vi "FPGA_RAPS.vi"(8 "error in":errorcluster) -> (0 "error out":errorcluster)   [LabVIEW 2010]
uses:
  fpgaVIsAndControls/DDS_board_init_cluster.ctl
  common_typedefs/channels_cluster.ctl
  fpgaVIsAndControls/FPGA_parameters_cluster.ctl
  common_typedefs/gate_parameters_cluster.ctl
  fpgaVIsAndControls/derived_values.ctl
  fpgaVIsAndControls/scan_point_cluster.ctl
  fpgaVIsAndControls/DDS_board_values_cluster.ctl
  fpgaVIsAndControls/synthesizer_point_cluster.ctl
  <vilib>/Platform/TimedLoop/XDataNode/XDataNode.xnode
  <vilib>/Platform/TimedLoop/XDataNode/timing_clust.ctl
  <vilib>/Platform/TimedLoop/XDataNode/nitl_modes.ctl
  <vilib>/Platform/TimedLoop/XDataNode/wakeup.ctl
  <vilib>/eio/EIONode/EIONode.xnode
  <vilib>/rvi/eio/nirviEIOImplementation/nirviEIOImplementation.xnode
  <vilib>/rvi/eio/common/nirviEmuClasses.ctl
  <vilib>/rvi/eio/nirviErrorMerge/nirviErrorMerge.xnode
  <vilib>/rvi/DataTransferAndStorage/Container/XNode/niFpgaContainer.xnode
  <vilib>/rvi/DataTransferAndStorage/Container/Common/niFpgaContainerMethod.ctl
  <vilib>/rvi/DataTransferAndStorage/Container/Common/niFpgaTransferTypeControl.ctl
  <vilib>/rvi/eio/common/nirviEmuTemplateMethod_noerrors.vi
  <vilib>/rvi/eio/common/nirviEmuTemplateMethod_errors.vi
  <vilib>/rvi/interface/RandomDataEmulation/nirviRandomDataFPGAFIFO.vi
  <vilib>/rvi/interface/RandomDataEmulation/niFpgaRandomDataHandleErrors.vi
  <vilib>/rvi/FIFO/Fifo_Resource/nirvififoEmulationSetSize.vi
  <vilib>/rvi/DataTransferAndStorage/Container/Common/niFpgaContainerGetUniqueNameForEmu.vi
  <vilib>/Platform/TimedLoop/XDataNode/XDNodeRunTimeDep.lvlib
panel:
  in  "shall acquisition start clocks?":bool
  in  "run clock 3":bool
  in  "run clock 2":bool
  in  "run clock 1":bool
  out "current memory pointer":i32
  in  "current raps point":T1
  out "current write address":u32
  in  "button:storePoint":bool
  out "current synthesizer point":T2
  out "current frequency point":T3
  out "current raps point":T1
  in  "point package size":u8=1
  out "derived values":T4={"AOD half bandwidth_x"=17500000.0, "AOD half bandwidth_y"=17500000.0, "x-point bandwidth"=10.0, "y-point bandwidth"=10.0} {"y-point bandwidth" format="%.28g"; "x-point bandwidth" format="%.28g"; "AOD half bandwidth_y" format="%.14g"; "AOD half bandwidth_x" format="%.14g"}
  out "next pixel?":bool
  in  "integration delay (iterations)":u32
  in  "integration delay (pixels)":u32
  in  "first pixel black?":bool
  in  "gate 1":T5
  in  "gate 2":T5
  in  "gate 3":T5
  out "clock 2 state":bool
  out "clock 1 state":bool
  out "clock 3 state":bool
  out "acquiring?":bool
  in  "in triggered mode?":bool
  in  "stop at FIFO overflow?":bool
  in  "converter box version":i16=1 min=1 max=2
  out "reset out":bool
  in  "ra trajectory pixels\n(data/pixels transfered)":u32=65535
  in  "amp comp":bool
  in  "inverse?":T6(ring)
  in  "OSK select":bool=TRUE
  in  "FPGA parameters":T7={"AOD Bandwidth_x (Hz)"=34000000.0, "AOD Bandwidth_y (Hz)"=34000000.0, "sin Phi"=0.0, "cos Phi"=1.0, "Bandwidth for LUTs (256pts)"=0.9999999999854481, "AOD_Amplitude in"=3400, "AOD center frequ. (Hz)_x"=94000000.0, "AOD center frequ. (Hz)_y"=94000000.0, "x offset (Hz)"=0.0, "y offset (Hz)"=0.0} {"AOD center frequ. (Hz)_y" format="%.14g"; "AOD center frequ. (Hz)_x" format="%.14g"; "cos Phi" format="%.35g"; "sin Phi" format="%.35g"}
  out "integrated pixel values":T8
  in  "maximum bit depth":i8=16
  in  "pixel iterations":u32=40
  in  "equilibration iterations":u32=200
  out "data read":T8
  in  "channel offsets":T8
  in  "number of pixels":i64=-1
  out "FIFO_DMA0 full?":bool
  out "current pixel no.":i64
  in  "acquire?":bool caption="Acquire?"
  in  "Stop complete VI":bool caption="Stop"
  in  "reset in":bool caption="Reset"
  in  "DDS board initialization parameters":T9={"Bypass PLL"=FALSE, "PLL Range"=TRUE, "Update Clock"=FALSE, "Triangle "=FALSE, "SDO Active"=FALSE, "LSB First"=FALSE, "OSK Int"=FALSE, "Output Shaped Keying Enable"=TRUE, "Bypass Sinc"=FALSE, "Digital Part"=TRUE, "OutPut DAC"=TRUE, "Control DAC"=TRUE, "Comparator"=FALSE, "Modus"=0, "Multiplier Value"=15} {"Modus" scale=0.0..4.0}
  # "FPGA integrator"
  # "IN"
  # "OUT"
  # "DDS"
  # "Clock parameters"
  # "DIO 1/32"
  # "PXI/RTSI 1"
  # "Store points"
  # "PXI/RTSI 2"
  # "FSK"
  # "Ramped"
  # "FSK"
  # "Chirp Modus"
  # "Unramped"
  # "BPSK"
  # "Single Tone"
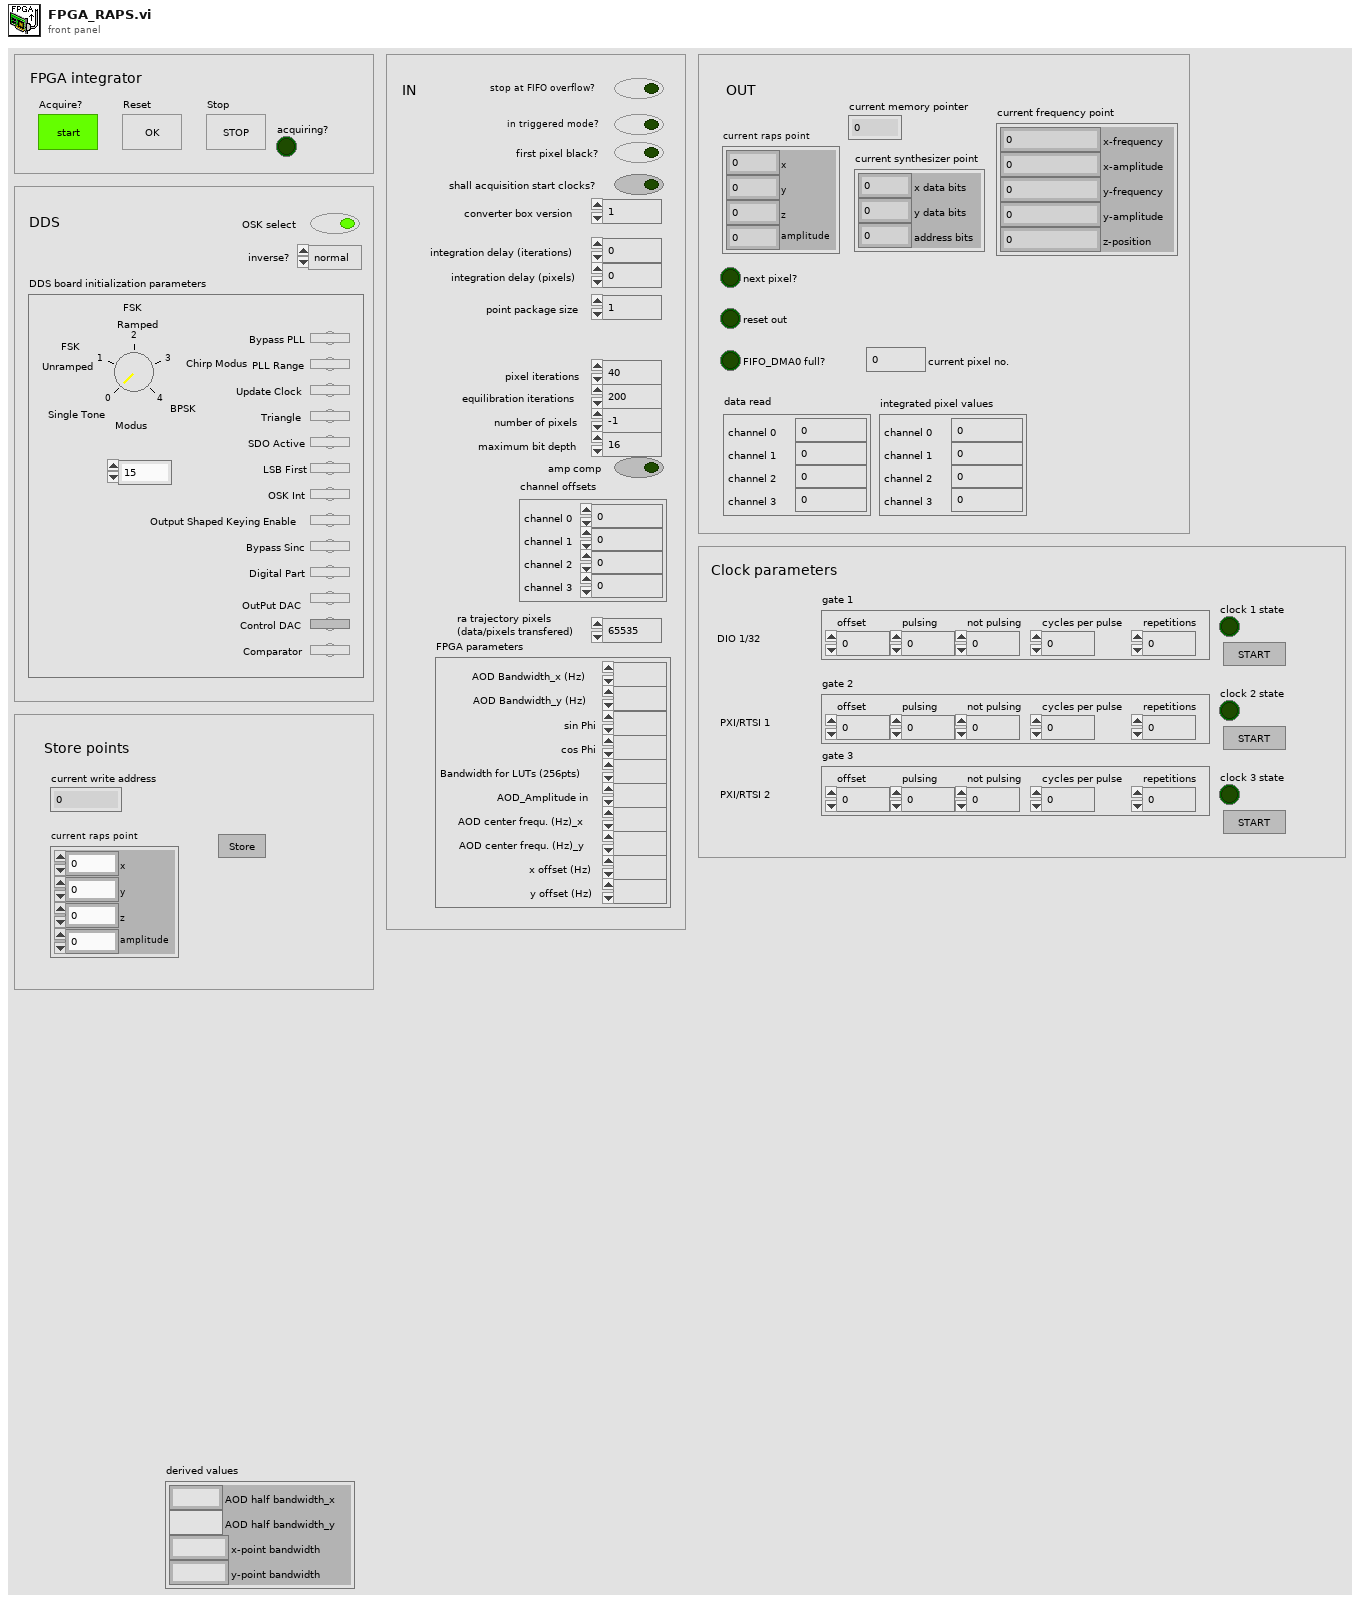
[diagram p1: front panel]
types:
  T1 = typedef "scan_point_cluster.ctl" = cluster{"x":u16, "y":u16, "z":u16, "amplitude":u16}
  T2 = typedef "synthesizer_point_cluster.ctl" = cluster{"x data bits":u8, "y data bits":u8, "address bits":u8}
  T3 = typedef "DDS_board_values_cluster.ctl" = cluster{"x-frequency":fxp<+/-,36,32>, "x-amplitude":u16, "y-frequency":fxp<+/-,36,32>, "y-amplitude":u16, "z-position":i16}
  T4 = typedef "derived_values.ctl" = cluster{"AOD half bandwidth_x":fxp<+/-,36,32>, "AOD half bandwidth_y":fxp<+/-,36,32>, "x-point bandwidth":fxp<+/-,36,32>, "y-point bandwidth":fxp<+/-,36,32>}
  T5 = typedef "gate_parameters_cluster.ctl" = cluster{"offset":i64, "pulsing":i64, "not pulsing":i64, "cycles per pulse":i64, "repetitions":i64}
  T6 = enum16{"normal", "x inversed", "y inversed", "x & y inversed"}
  T7 = typedef "FPGA_parameters_cluster.ctl" = cluster{"AOD Bandwidth_x (Hz)":fxp<+/-,36,32>, "AOD Bandwidth_y (Hz)":fxp<+/-,36,32>, "sin Phi":fxp<+/-,36,2>, "cos Phi":fxp<+/-,36,2>, "Bandwidth for LUTs (256pts)":fxp<+,36,0>, "AOD_Amplitude in":u16, "AOD center frequ. (Hz)_x":fxp<+/-,36,32>, "AOD center frequ. (Hz)_y":fxp<+/-,36,32>, "x offset (Hz)":fxp<+/-,36,32>, "y offset (Hz)":fxp<+/-,36,32>}
  T8 = typedef "channels_cluster.ctl" = cluster{"channel 0":u32, "channel 1":u32, "channel 2":u32, "channel 3":u32}
  T9 = typedef "DDS_board_init_cluster.ctl" = cluster{"Bypass PLL":bool, "PLL Range":bool, "Update Clock":bool, "Triangle ":bool, "SDO Active":bool, "LSB First":bool, "OSK Int":bool, "Output Shaped Keying Enable":bool, "Bypass Sinc":bool, "Digital Part":bool, "OutPut DAC":bool, "Control DAC":bool, "Comparator":bool, "Modus":u8, "Multiplier Value":u8}
  T10 = typedef "FPGA_constants_cluster.ctl" = cluster{"register":cluster{"Reg. 1D":u8, "Reg. 1E":u8, "Reg. 1F":u8, "Reg. 20":u8}}
  T11 = typedef "XDNodeRunTimeDep.lvlib/timing_clust.ctl" = cluster{"Expected End [f-1]":u64, "Actual End [f-1]":u64, "Finished Late? [f-1]":bool, "Expected End [i-1]":u64, "Actual End [i-1]":u64, "Finished Late? [i-1]":bool, "Expected Start [i]":u64, "Actual Start [i]":u64, "Expected Start [f]":u64, "Actual Start [f]":u64, "Source Name":string, "Structure Name":string, "Period":i64, "Deadline":i64, "Offset":i64, "Start":i64, "Priority":i32, "Timeout":i32, "Mode":T12, "Wakeup Reason":T13, "Error":errorcluster, "Source Type":string, "Secondary Source Type":string, "Global End Time":u64, "Global Start Time":u64, "Frame Duration":u64, "Iteration Duration":u64, "Assigned CPU":i32, "I/O Scan Engine Mode":u32}
  T12 = typedef "XDNodeRunTimeDep.lvlib/nitl_modes.ctl" = enum32{"No Change", "Process missed periods, maintain original phase", "Discard missed periods, maintain original phase", "Process missed periods, ignore original phase", "Discard missed periods, ignore original phase"}
  T13 = typedef "XDNodeRunTimeDep.lvlib/wakeup.ctl" = enum32{"Normal", "Aborted", "Asynchronous wakeup", "Timing source error", "Timed loop error", "Timeout"}
  T14 = typedef "nirviEmuClasses.ctl" = enum16{"IO Read", "IO Write", "Method", "Property Read", "Property Write"}
  T15 = typedef "niFpgaContainerMethod.ctl" = enum16{"<none>", "write", "read", "clear", "getNumberOfElementsToWrite", "getNumberOfElementsToRead", "enable", "disable", "flushAndDisable", "getStreamState", "readA", "readB", "dramWrite", "dramWriteWithByteEnables", "dramRequestData", "dramRetrieveData"}
  T16 = typedef "niFpgaTransferTypeControl.ctl" = enum16{"Target-Scoped", "Host to Target - DMA", "Target to Host - DMA", "Peer to Peer Reader", "Peer to Peer Writer", "Bidirectional"}
  T17 = typedef "gate_counters_cluster.ctl" = cluster{"phase iteration counter":i64, "phase repetition counter":i64, "pulse iteration counter":i64, "phase state":bool}
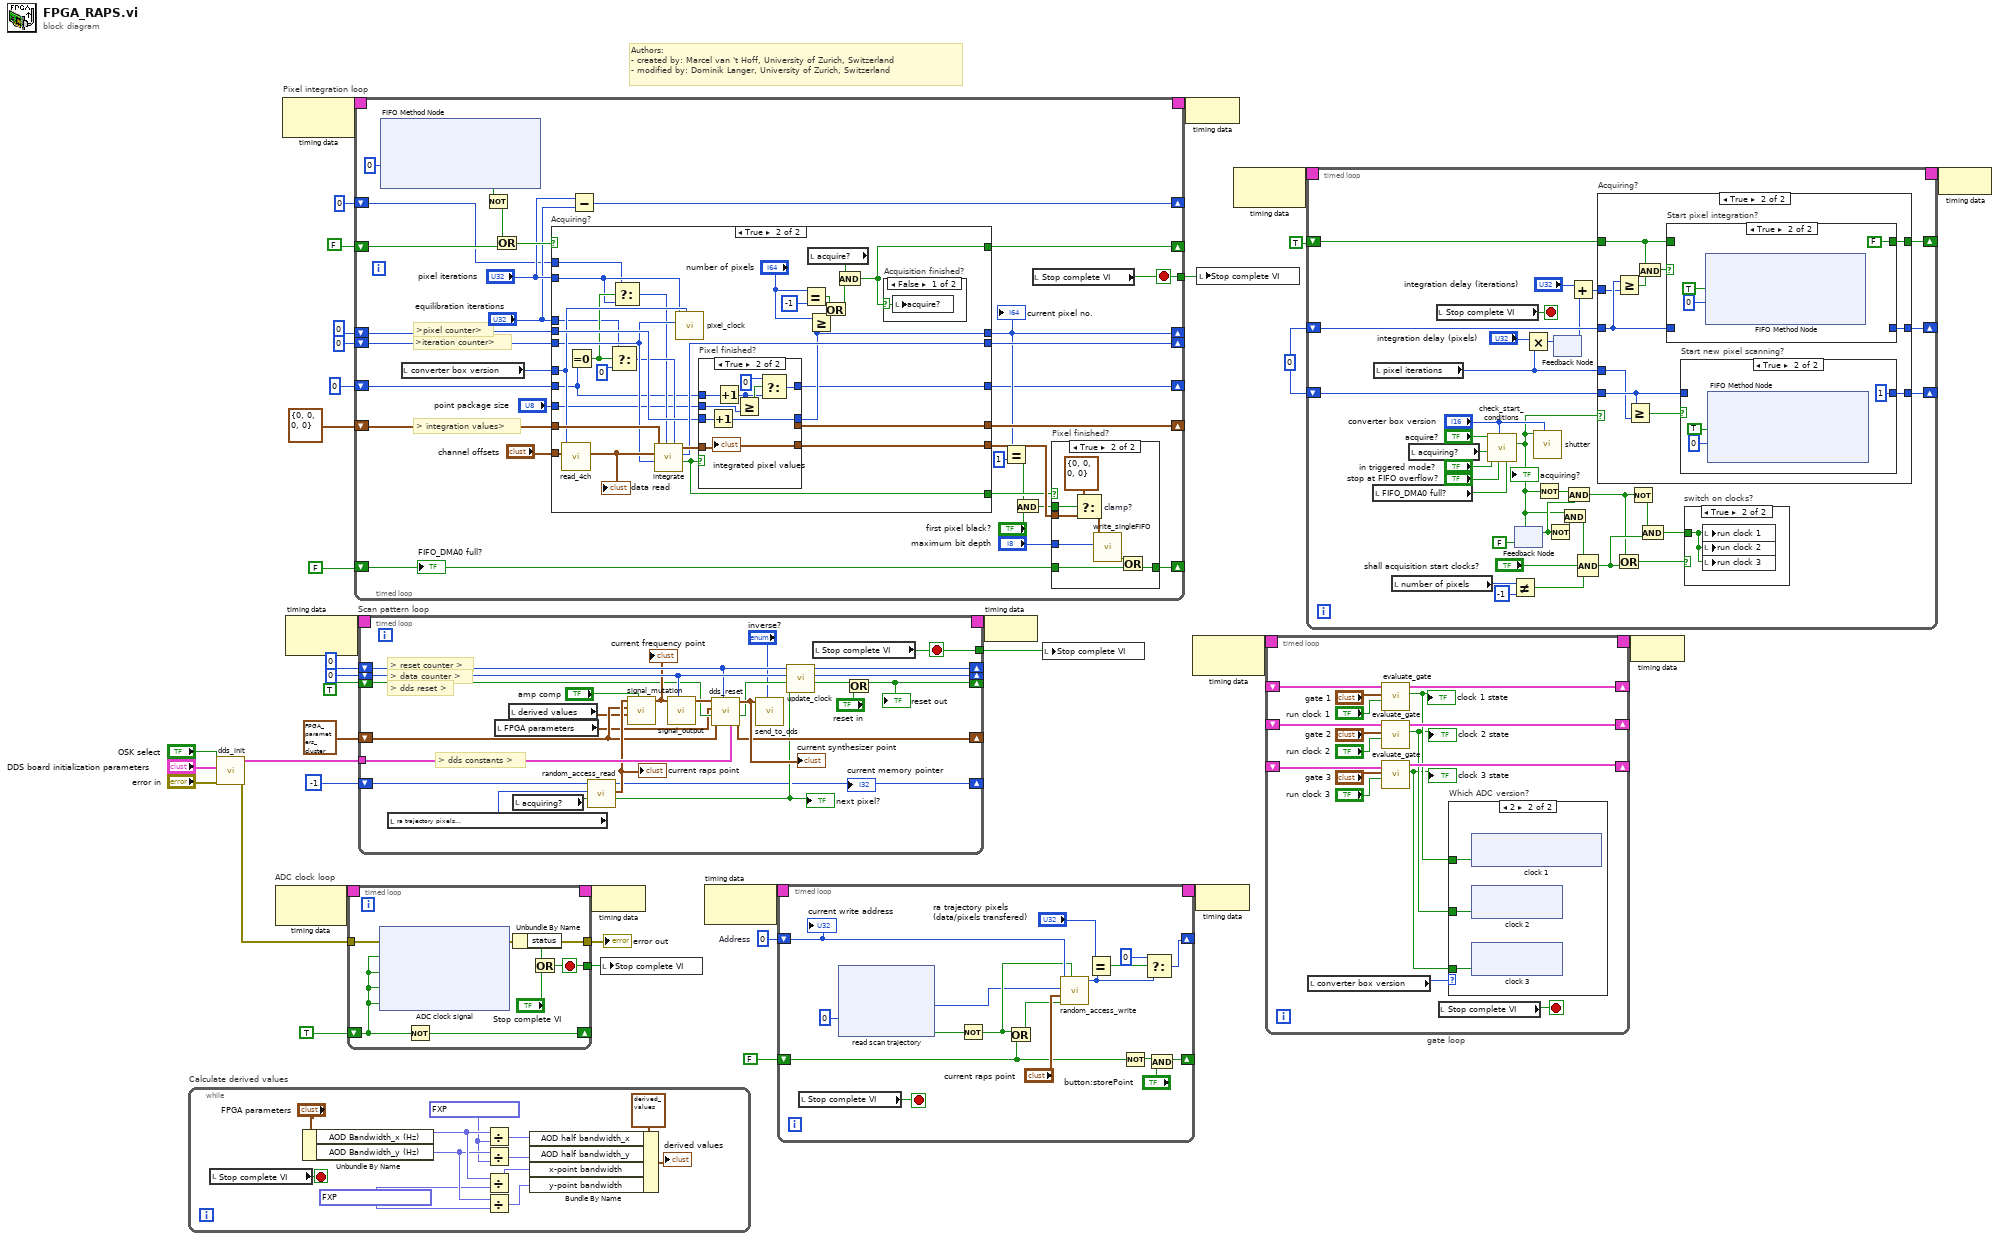
[diagram p0: block diagram]
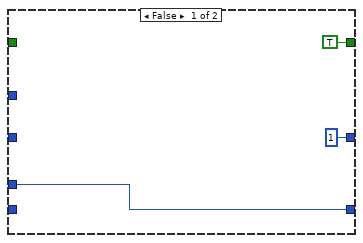
[diagram p3: hidden frame]
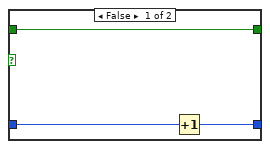
[diagram p4: hidden frame]
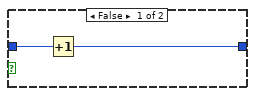
[diagram p5: hidden frame]
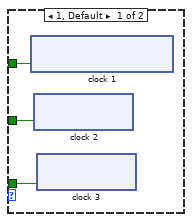
[diagram p6: hidden frame]
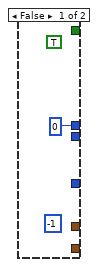
[diagram p8: hidden frame]
diagram:
  w8 = u32 0
  w14 = u32 0  # Address
  # "Authors: \n- created by: Marcel van 't Hoff, University of Zurich, Switzerland\n- modified by: Dominik Langer, University of Zurich, Switzerland"
  n1 = while "Calculate derived values" {
    stop <- w41 stop-if-true
    w42 = fxp<+/-,36,32> 2.0 ("y")
    w39 = fxp<+,36,32> 65534.0 ("y")
    n2 = local read "Stop complete VI"() -> (w41:bool)
    n3 = Unbundle By Name("FPGA parameters") -> ("AOD Bandwidth_x (Hz)"=w48:fxp<+/-,36,32>, "AOD Bandwidth_y (Hz)"=w47:fxp<+/-,36,32>)
    n4 = Divide(x=w48, y=w42) -> (x/y=w50:fxp<+/-,36,32>)
    n5 = Divide(x=w47, y=w42) -> (x/y=w49:fxp<+/-,36,32>)
    n6 = Divide(x=w48, y=w39) -> (x/y=w44:fxp<+/-,36,32>)
    n7 = Divide(x=w47, y=w39) -> (x/y=w43:fxp<+/-,36,32>)
    n8 = Bundle By Name(cluster=T4 {"AOD half bandwidth_x"=17500000.0, "AOD half bandwidth_y"=17500000.0, "x-point bandwidth"=10.0, "y-point bandwidth"=10.0} ("derived values"), "AOD half bandwidth_x"=w50, "AOD half bandwidth_y"=w49, "x-point bandwidth"=w44, "y-point bandwidth"=w43) -> (→"derived values":T4)
  }
  n9 = call "dds_init.vi"("error in"="error in", "DDS board initialization parameters"="DDS board initialization parameters", "OSK select"="OSK select") -> ("error out"=w32:errorcluster, "constants out"=w33:T10)  [unwired: 7 in]
  n10 = node-c288() -> (w38:T11)  [unwired: 1 out]
  n11 = node-c288() -> (w28:T11)  [unwired: 1 out]
  n12 = node-c288() -> (w25:T11)  [unwired: 1 in]
  n13 = timed-loop "ADC clock loop" {
    timing: w38 -> [_]
    timing-out: [_] -> w37
    shift-right: [w52] -> _
    shift-left: TRUE -> [w57]
    tunnel: [w54] -> w35
    tunnel: w32 -> [w53]
    tunnel: [w51] -> w22
    stop <- w54 stop-if-true
    n14 = xnode "ADC clock signal"("error in"=w53, "Connector0/DIO14"=w57, "Connector0/DIO15"=w57, "Connector1/DIO14"=w57, "Connector1/DIO15"=w57) -> ("error out"=w51:errorcluster)  [unwired: 4 in, 4 out]
    n15 = Not(x=w57) -> (.not. x?=w52:bool)
    n16 = Unbundle By Name(w51) -> ("status"=w55:bool)
    n17 = Or(x=w55, y="Stop complete VI") -> (x .or. y?=w54:bool)
  }
  "error out" <- w22
  n18 = timed-loop "Pixel integration loop" {
    timing: w28 -> [_]
    timing-out: [_] -> w27
    shift-right: [w185] -> _
    shift-left: T8 {"channel 0"=0, "channel 1"=0, "channel 2"=0, "channel 3"=0} ("channel offsets 2") -> [w184]
    shift-right: [w182] -> _
    shift-left: u32 0 ("iteration counter out") -> [w183]
    shift-right: [w164] -> _
    shift-left: i64 0 -> [w181]
    tunnel: [w180] -> w26
    shift-right: [w170] -> _
    shift-left: FALSE -> [w171]
    shift-right: [w172] -> _
    shift-left: FALSE -> [w174]
    shift-right: [w159] -> _
    shift-left: u8 0 ("f") -> [w161]
    shift-right: [w156] -> _
    shift-left: u32 0 -> [w155]
    stop <- w180 stop-if-true
    # ">pixel counter>"
    # "> integration values>"
    # ">iteration counter>"
    n19 = xnode ("FIFO Method Node")("Timeout"=0) -> ("Timed Out?"=w177:bool)  [unwired: 1 in, 2 out]
    n20 = local read "converter box version"() -> (w178:i16)
    n21 = Not(x=w177) -> (.not. x?=w175:bool)
    n22 = Or(x=w175, y=w174) -> (x .or. y?=w173:bool)
    n23 = case "Acquiring?" shown="True" w173 {
      tunnel: [_ w272] -> w185
      tunnel: w184 -> [_ w275]
      tunnel: [_ w261] -> w169
      tunnel: w183 -> [_ w259]
      tunnel: [_ w271] -> w182
      tunnel: w181 -> [_ w264]
      tunnel: [i64 0 w263] -> w164
      tunnel: "channel offsets" -> [_ w262]
      tunnel: "pixel iterations" -> [_ w254]
      tunnel: "equilibration iterations" -> [_ w253]
      tunnel: w178 -> [_ w260]
      tunnel: [_ w258] -> w172
      tunnel: [_ w257] -> w167
      tunnel: w161 -> [_ w248]
      tunnel: "point package size" -> [_ w249]
      tunnel: [_ w247] -> w159
      tunnel: w155 -> [_ w251]
      frame False {
        (unwired) -1 ("block index out")
        (unwired) TRUE
      }
      frame True {
        n24 = call "read_4ch.vi"("channel offsets"=w262, "converter box version"=w260) -> ("read output"=w273:T8)  [unwired: 9 in]
        "data read" <- w273
        n25 = Equal To 0?(x=w248) -> (x = 0?=w256:bool)
        n26 = Select(t=w253, s=w256, f=u32 0) -> (s? t:f=w255:u32)
        n27 = Select(t=w251, s=w256, f=w254) -> (s? t:f=w252:u32)
        n28 = call "integrate.vi"("waiting iterations per pixel"=w255, "integration iterations per pixel"=w252, "iteration counter in"=w259, "sampling values in"=w273, "previous pixel values in"=w275) -> ("finished?"=w257:bool, "iteration counter out"=w271:u32, "new pixel values out"=w274:T8)  [unwired: 4 in]
        n29 = call "pixel_clock.vi"("converter box version"=w260, "current iteration"=w259, "iterations per pixel"=w254) -> ()  [unwired: 9 in]
        n30 = case "Pixel finished?" shown="True" w257 {
          tunnel: w274 -> [w279 w286]
          tunnel: [w279 _] -> w272
          tunnel: [_ w286] -> w261
          tunnel: w264 -> [w278 w287]
          tunnel: [w278 w288] -> w263
          tunnel: w249 -> [_ w280]
          tunnel: w248 -> [w277 w281]
          tunnel: [w277 w282] -> w247
          frame False {
          }
          frame True {
            n31 = Increment(x=w287) -> (x+1=w288:i64)
            n32 = Increment(x=w281) -> (x+1=w283:u8)
            n33 = Greater Or Equal?(x=w283, y=w280) -> (x >= y?=w284:bool)
            n34 = Select(t=u8 0 ("f"), s=w284, f=w283) -> (s? t:f=w282:u8)
            "integrated pixel values" <- w286
          }
        }
        n35 = Equal?(x="number of pixels", y=i64 -1 ("x")) -> (x = y?=w268:bool)
        n36 = Greater Or Equal?(x="number of pixels", y=w263) -> (x >= y?=w267:bool)
        n37 = local read "acquire?"() -> (w270:bool)
        n38 = Or(x=w268, y=w267) -> (x .or. y?=w269:bool)
        n39 = And(x=w270, y=w269) -> (x .and. y?=w258:bool)
        n40 = case "Acquisition finished?" shown="False" w258 {
          selector: w258 -> [w276 _]
          frame False {
            n41 = local write "acquire?"(w276) -> ()
          }
          frame True {
          }
        }
      }
    }
    "current pixel no." <- w164
    n42 = Subtract(x="pixel iterations", y="equilibration iterations") -> (x-y=w156:u32)
    n43 = Equal?(x=w164, y=i64 1) -> (x = y?=w166:bool)
    n44 = And(x=w166, y="first pixel black?") -> (x .and. y?=w162:bool)
    n45 = local read "Stop complete VI"() -> (w180:bool)
    n46 = case "Pixel finished?" shown="True" w167 {
      tunnel: w171 -> [w186 w193]
      tunnel: [w186 w192] -> w170
      tunnel: w169 -> [_ w190]
      tunnel: "maximum bit depth" -> [_ w188]
      tunnel: w162 -> [_ w187]
      frame False {
      }
      frame True {
        n47 = Select "clamp?"(t=T8 {"channel 0"=0, "channel 1"=0, "channel 2"=0, "channel 3"=0}, s=w187, f=w190) -> (s? t:f=w189:T8)
        n48 = call "write_singleFIFO.vi"("maximum bit depth"=w188, "values to be written"=w189) -> ("FIFO overflow"=w194:bool)  [unwired: 9 in]
        n49 = Or(x=w194, y=w193) -> (x .or. y?=w192:bool)
      }
    }
    "FIFO_DMA0 full?" <- w171
  }
  n50 = timed-loop "Scan pattern loop" {
    tunnel: [w305] -> w34
    tunnel: w33 -> [w310]
    shift-right: [w307] -> _
    shift-left: T7 {"AOD Bandwidth_x (Hz)"=35000000.0, "AOD Bandwidth_y (Hz)"=35000000.0, "sin Phi"=1.9999999999417923, "cos Phi"=1.9999999999417923, "Bandwidth for LUTs (256pts)"=0.0, "AOD_Amplitude in"=0, "AOD center frequ. (Hz)_x"=1.0, "AOD center frequ. (Hz)_y"=0.0, "x offset (Hz)"=1.0, "y offset (Hz)"=0.0} ("FPGA parameters out 2") -> [w302]
    shift-right: [w315] -> _
    shift-left: TRUE ("reset dds out") -> [w299]
    shift-right: [w314] -> _
    shift-left: u32 0 ("data sending counter (#bytes) out") -> [w313]
    shift-right: [w312] -> _
    shift-left: u8 0 ("reset counter out") -> [w309]
    timing: w25 -> [_]
    timing-out: [_] -> w24
    shift-right: [w291] -> _
    shift-left: -1 ("scan points cluster out") -> [w292]
    stop <- w305 stop-if-true
    # "> dds constants >"
    # "> dds reset >"
    # "> data counter >"
    # "> reset counter >"
    n51 = local read "ra trajectory pixels\n(data/pixels transfered)"() -> (w294:u32)
    n52 = local read "FPGA parameters"() -> (w295:T7)
    n53 = local read "derived values"() -> (w296:T4)
    n54 = local read "acquiring?"() -> (w293:bool)
    n55 = call "random_access_read.vi"("ra scanning?"=w293, "number of points"=w294, "memory pointer in"=w292) -> ("new pixel update?"=w304:bool, "raps point"=w303:T1, "memory pointer out"=w291:i32)  [unwired: 6 in]
    "next pixel?" <- w304
    "current raps point" <- w303
    "current memory pointer" <- w291
    n56 = call "signal_mutation.vi"("amplitude compensation?"="amp comp", "derived values"=w296, "FPGA parameters"=w302, "point"=w303) -> ("frequency point"=w301:T3)  [unwired: 7 in]
    "current frequency point" <- w301
    n57 = call "signal_output.vi"("pipeline counter in"=w313, "frequency point"=w301) -> ("synthesizer point"=w300:T2)  [unwired: 9 in]
    n58 = call "dds_reset.vi"("constants in"=w310, "counter in"=w309, "FPGA parameters in"=w302, "reset dds in"=w299, "FPGA parameters after reset"=w295, "synthesizer point in"=w300) -> ("FPGA parameters out"=w307:T7, "reset dds out"=w298:bool, "synthesizer point out"=w316:T2)  [unwired: 3 in]
    "current synthesizer point" <- w316
    n59 = call "send_to_dds.vi"("inversion selector"="inverse?", "synthesizer point"=w316) -> ()  [unwired: 10 in]
    n60 = call "update_clock.vi"("update command in"=w304, "update reset counter in"=w298, "data sending counter (#bytes) in"=w313, "reset counter in"=w309) -> ("update reset counter out"=w308:bool, "data sending counter (#bytes) out"=w314:u32, "reset counter out"=w312:u8)  [unwired: 5 in]
    n61 = local read "Stop complete VI"() -> (w305:bool)
    n62 = Or(x=w308, y="reset in") -> (x .or. y?=w315:bool)
    "reset out" <- w315
  }
  n63 = node-c288(w37) -> ()
  n64 = local write "Stop complete VI"(w35) -> ()
  n65 = node-c288() -> (w16:T11)  [unwired: 1 in]
  n66 = timed-loop {
    timing: w16 -> [_]
    timing-out: [_] -> w15
    shift-right: [w330] -> _
    shift-left: w14 -> [w334]
    shift-right: [w326] -> _
    shift-left: FALSE -> [w321]
    stop <- w333 stop-if-true
    n67 = local read "Stop complete VI"() -> (w333:bool)
    n68 = xnode "read scan trajectory"("Timeout"=0) -> ("Element"=w322:u64, "Timed Out?"=w325:bool)  [unwired: 1 in, 1 out]
    n69 = Not(x=w325) -> (.not. x?=w323:bool)
    n70 = Or(x=w323, y=w321) -> (x .or. y?=w320:bool)
    n71 = call "random_access_write.vi"("is encoded point?"=w323, "write?"=w320, "raps point"="current raps point", "encoded point"=w322, "address in"=w334) -> ("address out"=w331:u32)  [unwired: 6 in]
    n72 = Equal?(x="ra trajectory pixels\n(data/pixels transfered)", y=w331) -> (x = y?=w332:bool)
    n73 = Not(x=w321) -> (.not. x?=w327:bool)
    n74 = Select(t=u32 0, s=w332, f=w331) -> (s? t:f=w330:u32)
    n75 = And(x=w327, y="button:storePoint") -> (x .and. y?=w326:bool)
    "current write address" <- w334
  }
  n76 = node-c288(w24) -> ()
  n77 = local write "Stop complete VI"(w34) -> ()
  n78 = node-c288(w27) -> ()
  n79 = node-c288() -> (w13:T11)  [unwired: 1 in]
  n80 = node-c288(w15) -> ()
  n81 = local write "Stop complete VI"(w26) -> ()
  n82 = node-c288() -> (w10:T11)  [unwired: 1 in]
  n83 = timed-loop "gate loop" {
    timing: w13 -> [_]
    timing-out: [_] -> w12
    shift-right: [w382] -> _
    shift-left: _ -> [w383]
    shift-right: [w380] -> _
    shift-left: _ -> [w381]
    shift-right: [w379] -> _
    shift-left: _ -> [w378]
    stop <- w370 stop-if-true
    n84 = local read "converter box version"() -> (w371:i16)
    n85 = call "evaluate_gate.vi"("acquiring?"="run clock 1", "gate settings"="gate 1", "gate counters in"=w383) -> ("pulse state out"=w374:bool, "gate counters out"=w382:T17)  [unwired: 7 in]
    "clock 1 state" <- w374
    n86 = call "evaluate_gate.vi"("acquiring?"="run clock 2", "gate settings"="gate 2", "gate counters in"=w381) -> ("pulse state out"=w373:bool, "gate counters out"=w380:T17)  [unwired: 7 in]
    "clock 2 state" <- w373
    n87 = call "evaluate_gate.vi"("acquiring?"="run clock 3", "gate settings"="gate 3", "gate counters in"=w378) -> ("pulse state out"=w372:bool, "gate counters out"=w379:T17)  [unwired: 7 in]
    "clock 3 state" <- w372
    n88 = local read "Stop complete VI"() -> (w370:bool)
    n89 = case "Which ADC version?" shown="2" w371 {
      tunnel: w374 -> [w384 w422]
      tunnel: w373 -> [w385 w421]
      tunnel: w372 -> [w386 w420]
      frame 1, Default {
        n90 = xnode "clock 1"("Connector1/DIO32"=w384) -> ()  [unwired: 1 in, 1 out]
        n91 = xnode "clock 2"("PXI_RTSI_1"=w385) -> ()  [unwired: 1 in, 1 out]
        n92 = xnode "clock 3"("PXI_RTSI_2"=w386) -> ()  [unwired: 1 in, 1 out]
      }
      frame 2 {
        n93 = xnode "clock 1"("Connector0/DIO38"=w422) -> ()  [unwired: 1 in, 1 out]
        n94 = xnode "clock 2"("PXI_RTSI_1"=w421) -> ()  [unwired: 1 in, 1 out]
        n95 = xnode "clock 3"("PXI_RTSI_2"=w420) -> ()  [unwired: 1 in, 1 out]
      }
    }
  }
  n96 = timed-loop {
    timing: w10 -> [_]
    timing-out: [_] -> w9
    shift-right: [w489] -> _
    shift-left: w8 -> [w490]
    shift-right: [w487] -> _
    shift-left: w8 -> [w488]
    shift-right: [w479] -> _
    shift-left: TRUE -> [w480]
    stop <- w491 stop-if-true
    n97 = local read "FIFO_DMA0 full?"() -> (w486:bool)
    n98 = local read "pixel iterations"() -> (w473:u32)
    n99 = local read "number of pixels"() -> (w460:i64)
    n100 = local read "acquiring?"() -> (w481:bool)
    n101 = local read "Stop complete VI"() -> (w491:bool)
    n102 = call "check_start_conditions.vi"("FIFO overflow?"=w486, "stop at FIFO overflow?"="stop at FIFO overflow?", "converter box version"="converter box version", "already acquiring?"=w481, "in triggered mode?"="in triggered mode?", "acquire"="acquire?") -> ("acquire?"=w462:bool)  [unwired: 5 in]
    "acquiring?" <- w462
    n103 = Not Equal?(x=w460, y=i64 -1 ("x")) -> (x != y?=w471:bool)
    n104 = feedback #1(FALSE ("acquire?")) -> (w466:bool)
    n105 = feedback-in #1(w462) -> ()
    n106 = Multiply(x="integration delay (pixels)", y=w473) -> (x*y=w475:u32)
    n107 = call "shutter.vi"("converter box version"="converter box version", "open?"=w462) -> ()  [unwired: 10 in]
    n108 = Not(x=w462) -> (.not. x?=w470:bool)
    n109 = Not(x=w466) -> (.not. x?=w468:bool)
    n110 = feedback-in #2(w475) -> ()
    n111 = feedback #2() -> (w474:u32)  [unwired: 1 in]
    n112 = And(x=w462, y=w468) -> (x .and. y?=w467:bool)
    n113 = And(x=w470, y=w466) -> (x .and. y?=w463:bool)
    n114 = Add(x="integration delay (iterations)", y=w474) -> (x+y=w476:u32)
    n115 = Compound Arithmetic op=AND(w467, "shall acquisition start clocks?", w471) -> (w465:bool)
    n116 = case "Acquiring?" shown="True" w462 {
      tunnel: w490 -> [_ w503]
      tunnel: [w495 w505] -> w489
      tunnel: w488 -> [_ w500]
      tunnel: [u32 1 w504] -> w487
      tunnel: w473 -> [w495 w502]
      tunnel: w480 -> [_ w496]
      tunnel: [TRUE w501] -> w479
      tunnel: w476 -> [_ w499]
      frame False {
      }
      frame True {
        n117 = Greater Or Equal?(x=w500, y=w499) -> (x >= y?=w498:bool)
        n118 = Greater Or Equal?(x=w503, y=w502) -> (x >= y?=w506:bool)
        n119 = And(x=w496, y=w498) -> (x .and. y?=w497:bool)
        n120 = case "Start pixel integration?" shown="True" w497 {
          tunnel: w500 -> [w509 _]
          tunnel: [w508 _] -> w504
          tunnel: w496 -> [w507 _]
          tunnel: [w507 FALSE] -> w501
          frame False {
            n121 = Increment(x=w509) -> (x+1=w508:u32)
          }
          frame True {
            n122 = xnode ("FIFO Method Node")("Element"=TRUE, "Timeout"=0) -> ()  [unwired: 1 in, 2 out]
          }
        }
        n123 = case "Start new pixel scanning?" shown="True" w506 {
          tunnel: w503 -> [w565 _]
          tunnel: [w564 u32 1] -> w505
          frame False {
            n124 = Increment(x=w565) -> (x+1=w564:u32)
          }
          frame True {
            n125 = xnode ("FIFO Method Node")("Element"=TRUE, "Timeout"=0) -> ()  [unwired: 1 in, 2 out]
          }
        }
      }
    }
    n126 = Or(x=w463, y=w465) -> (x .or. y?=w459:bool)
    n127 = Not(x=w463) -> (.not. x?=w464:bool)
    n128 = And(x=w464, y=w465) -> (x .and. y?=w458:bool)
    n129 = case "switch on clocks?" shown="True" w459 {
      tunnel: w458 -> [_ w492]
      frame False {
      }
      frame True {
        n130 = local write "run clock 1"(w492) -> ()
        n131 = local write "run clock 2"(w492) -> ()
        n132 = local write "run clock 3"(w492) -> ()
      }
    }
  }
  n133 = node-c288(w12) -> ()
  n134 = node-c288(w9) -> ()
